vi "Calibration-SH.vi"(8 "Error In":errorcluster) -> (0 "Error Out":errorcluster, 2 "Offset":dbl, 3 "Gain":dbl)   [LabVIEW 2020, in "CollectionSupport.lvlib"]
uses:
  CollectionSupport.lvlib
  <vilib>/express/express shared/transition.llb/Dynamic To Waveform Array.vi
  <vilib>/express/express arith-compare/Formula/Block/exnFormulaBlock how many pts in the wave.vi
  <vilib>/express/express shared/ex_Modify Signal Name.vi
  <vilib>/express/express shared/transition.llb/Waveform Array To Dynamic.vi
  <vilib>/express/express arith-compare/Formula/XNode/ExpressFormulaBlockNode.xnode
panel:
  out "Message":string
  out "Pressure":dbl[](array[numeric])
  out "Flow":dbl[](array[numeric])
  out "XY Graph":cluster{"Y":dbl[], "Y":dbl[]}[](graph)
  in  "File Path":path
  in  "Flow":dbl
  in  "Save?":bool
  out "Pressure":dbl format="%.4f"
  out "Chart":dynamicdata(graph)
  in  "Add":bool
  in  "stop (F)":bool caption="Stop (F)"
  # "Flow"
  # "Pressure"
  # "Calculated Gain"
  # "Offset"
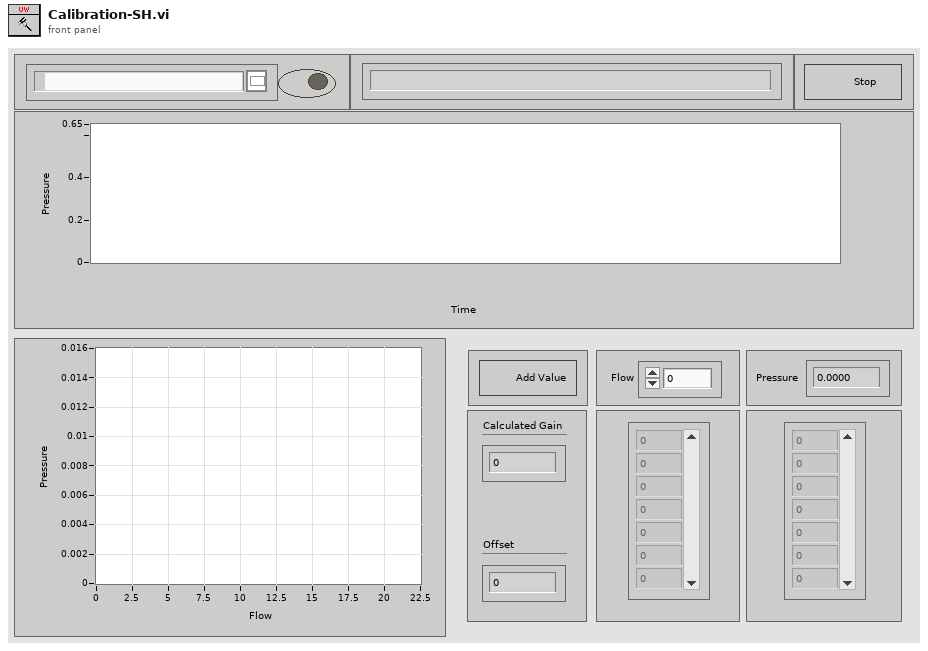
[diagram p1: front panel]
types:
  T1 = enum16{"open", "replace", "create", "open or create", "replace or create", "replace or create with confirmation"}
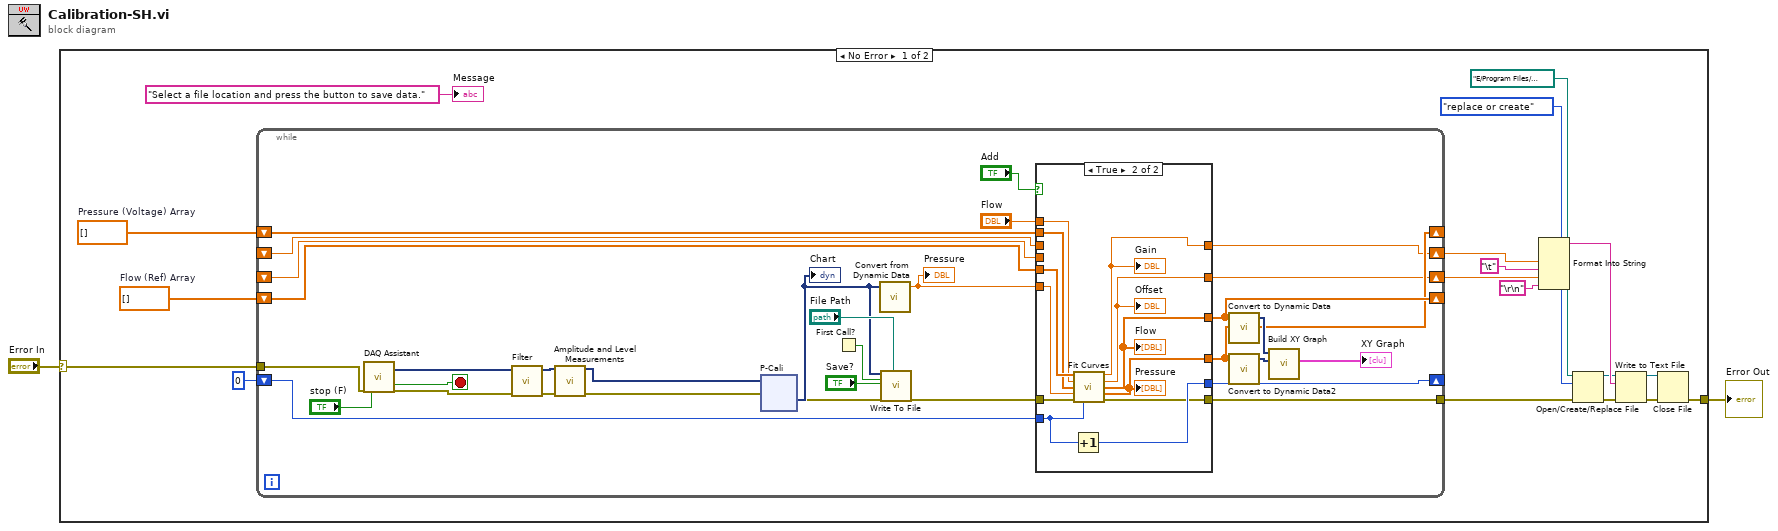
[diagram p0: block diagram]
diagram:
  n1 = case shown="No Error" "Error In" {
    selector: "Error In" -> [w3 w210]
    tunnel: [w11 w210] -> w1
    frame No Error {
      w18 = dbl[] []  # Pressure (Voltage) Array
      w20 = dbl[] []  # Flow (Ref) Array
      n2 = while {
        tunnel: w3 -> [w52]
        shift-right: [w42] -> _
        shift-left: w20 -> [w36]
        shift-right: [w41] -> _
        shift-left: w18 -> [w35]
        shift-right: [w39] -> _
        shift-left: 0 ("index") -> [w40]
        tunnel: [w34] -> w10
        shift-right: [w33] -> w5
        shift-left: _ -> [w31]
        shift-right: [w32] -> w4
        shift-left: _ -> [w30]
        stop <- w50 stop-if-true
        n3 = call "DAQ Assistant"("error in"=w52, "stop (F)"="stop (F)") -> ("data"=w28:dynamicdata, "stopped"=w50:bool, "error out"=w29:errorcluster)  [unwired: 14 in, 1 out]
        n4 = call "Filter"("error in (no error)"=w29, "Signal"=w28) -> ("error out"=w26:errorcluster, "Filtered Signal"=w25:dynamicdata)  [unwired: 8 in]
        n5 = call "Amplitude and Level Measurements"("Signals"=w25, "error in (no error)"=w26) -> ("Mean (DC)"=w21:dynamicdata, "error out"=w22:errorcluster)  [unwired: 12 in]
        n6 = xnode "P-Cali"("V"=w21, "error in (no error)"=w22) -> ("Result"=w27:dynamicdata, "error out"=w24:errorcluster)
        "Chart" <- w27
        n7 = First Call?() -> (First Call?: T/F=w48:bool)
        n8 = call "Convert from Dynamic Data"("Dynamic Data Type"=w27) -> ("Scalar"=w23:dbl)  [unwired: 3 in]
        "Pressure" <- w23
        n9 = call "Write To File"("Signals"=w27, "Reset"=w48, "Enable"="Save?", "error in (no error)"=w24, "Filename"="File Path") -> ("error out"=w37:errorcluster)  [unwired: 12 in, 2 out]
        n10 = case shown="True" "Add" {
          tunnel: "Flow" -> [_ w204]
          tunnel: [w197 w201] -> w42
          tunnel: [w196 w200] -> w41
          tunnel: w35 -> [w196 w203]
          tunnel: w36 -> [w197 w205]
          tunnel: w40 -> [w195 w208]
          tunnel: [w195 w209] -> w39
          tunnel: w37 -> [w194 w207]
          tunnel: [w194 w206] -> w34
          tunnel: w23 -> [_ w202]
          tunnel: [w193 w199] -> w33
          tunnel: [w192 w198] -> w32
          tunnel: w31 -> [w193 _]
          tunnel: w30 -> [w192 _]
          frame False {
          }
          frame True {
            n11 = Increment(x=w208) -> (x+1=w209:i32)
            n12 = call "Fit Curves.vi"("Reference (Array)"=w205, "Reference (Value)"=w204, "Voltage (Array)"=w203, "Voltage (Value)"=w202, "Error In"=w207, "index"=w208) -> ("Slope"=w199:dbl, "Intercept"=w198:dbl, "Reference Out"=w201:dbl[], "Voltage Out"=w200:dbl[], "Error Out"=w206:errorcluster)  [unwired: 5 in]
            "Gain" <- w199
            "Offset" <- w198
            "Flow" <- w201
            "Pressure" <- w200
          }
        }
        n13 = call "Convert to Dynamic Data"("Array"=w42) -> ("Dynamic Data Type"=w44:dynamicdata)  [unwired: 3 in]
        n14 = call "Convert to Dynamic Data2"("Array"=w41) -> ("Dynamic Data Type"=w43:dynamicdata)  [unwired: 3 in]
        n15 = call "Build XY Graph"("Y Input"=w43, "X Input"=w44) -> ("XY Graph"=→"XY Graph":cluster{"Y":dbl[], "Y":dbl[]}[])  [unwired: 8 in, 1 out]
      }
      n16 = Format Into String(w5, "\t", w4, "\r\n") -> (resulting string=w14:string)  [unwired: 3 in, 1 out]
      n17 = Open/Create/Replace File(file path (use dialog)=path "E:/Program Files/Master Aero Program/Calibration .txt files/SH Cali.txt", error in=w10, operation (0:open)=T1."replace or create") -> (refnum out=w12:refnum<file>, error out=w15:errorcluster)  [unwired: 3 in, 1 out]
      n18 = Write to Text File(file (use dialog)=w12, text=w14, error in=w15) -> (refnum out=w13:refnum<file>, error out=w16:errorcluster)  [unwired: 1 in, 1 out]
      n19 = Close File(refnum=w13, error in=w16) -> (error out=w11:errorcluster)  [unwired: 1 out]
      "Message" <- "Select a file location and press the button to save data." ("Message")
    }
    frame Error {
    }
  }
  "Error Out" <- w1
